vi "HeaderAction.vi"(0 "OR77200 en entrée":refnum<class "OR77200.lvclass"> caption="DNL_LabVIEW Object in", 11 "error in (no error)":errorcluster caption="entrée d'erreur (pas d'erreur)") -> (4 "OR77200 en sortie":refnum<class "OR77200.lvclass"> caption="DNL_LabVIEW Object out", 6 "DataNames":string[](array[string]), 8 "Instr Name":string, 10 "HeaderString":string, 14 "DisplayNames":string[](array[string]), 15 "error out":errorcluster caption="sortie d'erreur")   [LabVIEW 2012, in "OR77200.lvclass"]
uses:
  OR77200.lvclass
  OR77200.lvclass/OR77200.ctl
  BaseDevice/BaseDevice.lvclass
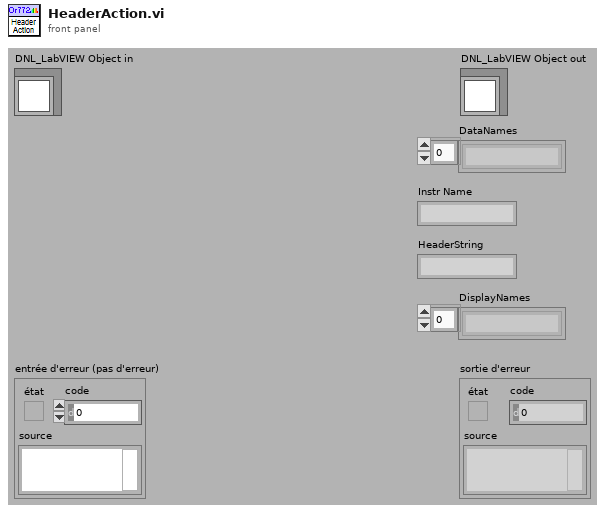
[diagram p1: front panel]
types:
  T1 = typedef "OR77200.lvclass/OR77200_Func.ctl" = enum16{"Position (nm)"}
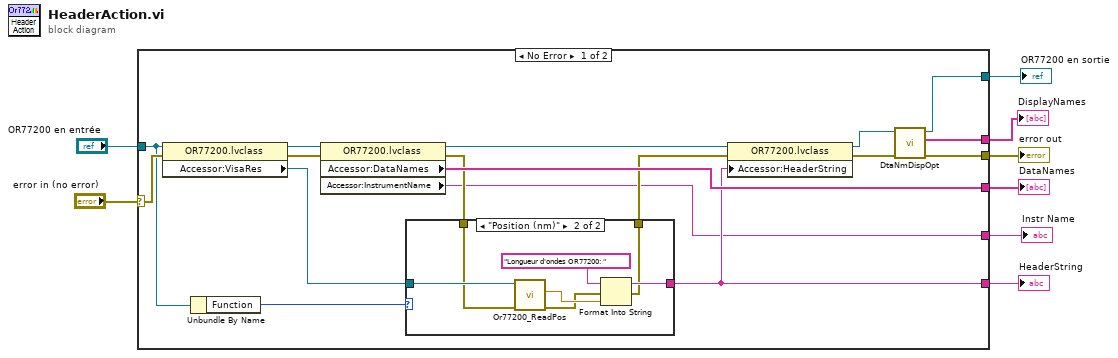
[diagram p0: block diagram]
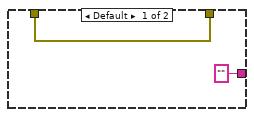
[diagram p2: hidden frame]
diagram:
  n1 = case shown="No Error" "error in (no error)" {
    selector: "error in (no error)" -> [w22 w35]
    tunnel: "OR77200 en entrée" -> [w16 w36]
    tunnel: [w11 w36] -> w6
    tunnel: [w24 _] -> w5
    tunnel: [w18 _] -> w4
    tunnel: [w12 w35] -> w3
    tunnel: [w14 _] -> w2
    tunnel: [w9 _] -> w1
    frame No Error {
      n2 = property class="OR77200.lvclass"(reference=w16, error in=w22) -> (reference out=w23:refnum<class "OR77200.lvclass">, error out=w20:errorcluster, "Accessor:VisaRes"=w21:refnum<visa-resource-name>)
      n3 = Unbundle By Name(w16) -> ("Function"=w15:T1)
      n4 = property class="OR77200.lvclass"(reference=w23, error in=w20) -> (reference out=w25:refnum<class "OR77200.lvclass">, error out=w19:errorcluster, "Accessor:DataNames"=w24:string[], "Accessor:InstrumentName"=w14:string)
      n5 = case shown="\"Position (nm)\"" w15 {
        tunnel: w21 -> [_ w34]
        tunnel: w19 -> [w26 w30]
        tunnel: ["" w29] -> w18
        tunnel: [w26 w28] -> w17
        frame Default {
        }
        frame "Position (nm)" {
          n6 = call <userlib>:"Or77200_ReadPos.vi"("error In"=w30, "Port"=w34) -> ("sortie d'erreur"=w31:errorcluster, "Lambda Out (nm)"=w33:dbl)  [unwired: 7 in, 1 out]
          n7 = Format Into String(initial string="Longueur d'ondes OR77200: ", error in=w31, w33) -> (resulting string=w29:string, error out=w28:errorcluster)  [unwired: 1 in]
        }
      }
      n8 = property class="OR77200.lvclass"(reference=w25, error in=w17, "Accessor:HeaderString"=w18) -> (reference out=w10:refnum<class "OR77200.lvclass">, error out=w13:errorcluster)
      n9 = call "DtaNmDispOpt.vi"("error in (no error)"=w13, "BaseDevice en entrée"=w10) -> ("error out"=w12:errorcluster, "DisplayNames"=w9:string[], "BaseDevice en sortie"=w11:refnum<class "OR77200.lvclass">)  [unwired: 7 in]
    }
    frame Error {
    }
  }
  "error out" <- w3
  "OR77200 en sortie" <- w6
  "DataNames" <- w5
  "HeaderString" <- w4
  "Instr Name" <- w2
  "DisplayNames" <- w1
